vi "Fetch Array (Voltage).vi"(0 "VISA resource name":refnum<visa-resource-name>, 11 "error in (no error)":errorcluster) -> (4 "VISA resource name out":refnum<visa-resource-name>, 6 "Samples (V)":dbl[](array[numeric]), 15 "error out":errorcluster)   [LabVIEW 2012, in "NH Research Regenerative Test Series.lvlib"]
doc: "Return an array containing the instantaneous input voltage in Volts. Query Number of Samples is called internally to read how many samples are available to read from the instruments buffer.\n\nWaveforms are captured with every initiated measurement based on the Set Aperture Length.vi and Set Number of Samples.vi commands. A measurement must be initiated first using a Read command or calling Initiate Measurement.vi."
uses:
  <instrlib>/NH Research Regenerative Test Series/NH Research Regenerative Test Series.lvlib
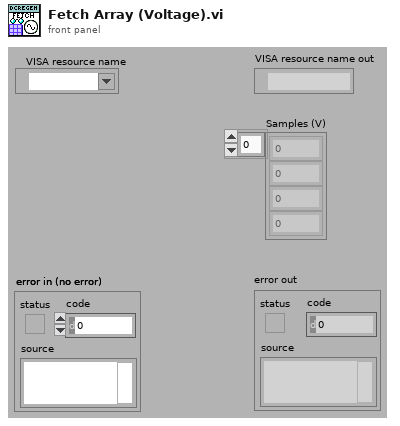
[diagram p1: front panel]
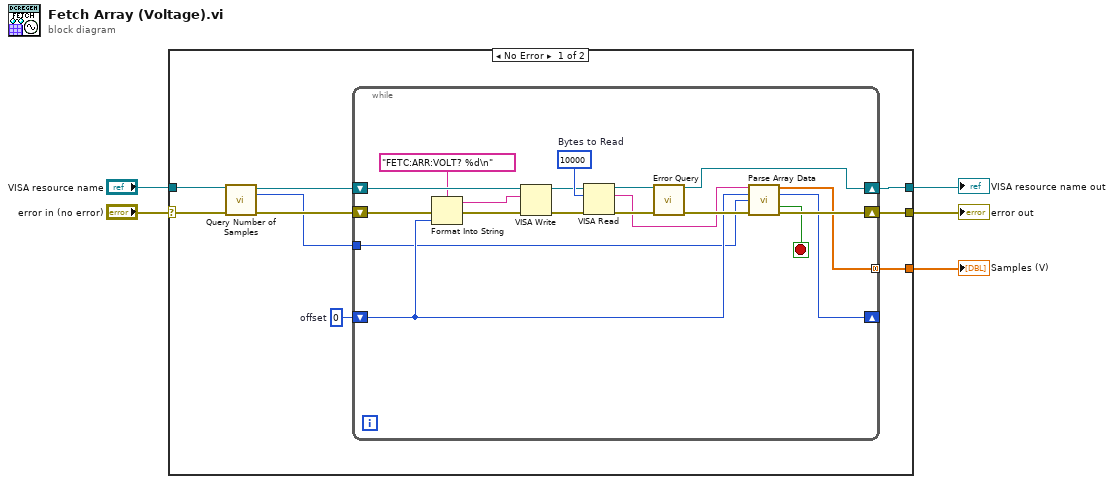
[diagram p0: block diagram]
diagram:
  n1 = case shown="No Error" "error in (no error)" {
    selector: "error in (no error)" -> [w10 w35]
    tunnel: [w13 w35] -> w4
    tunnel: [w14 w34] -> w1
    tunnel: "VISA resource name" -> [w9 w34]
    tunnel: [w12 _] -> w2
    frame No Error {
      w11 = 0  # offset
      n2 = call <instrlib>:"Query Number of Samples.vi"("VISA resource name"=w9, "error in (no error)"=w10) -> ("VISA resource name out"=w8:refnum<visa-resource-name>, "Number of Samples"=w6:u32, "error out"=w7:errorcluster)  [unwired: 11 in]
      n3 = while {
        shift-right: [w22] -> w13
        shift-left: w7 -> [w26]
        shift-right: [w15] -> w14
        shift-left: w8 -> [w30]
        tunnel: [w17] -> w12 mode=concatenating
        shift-right: [w18] -> _
        shift-left: w11 -> [w20]
        tunnel: w6 -> [w19]
        stop <- w16 stop-if-true
        w33 = u32 10000  # Bytes to Read
        n4 = Format Into String(format string="FETC:ARR:VOLT? %d\n", error in=w26, w20) -> (resulting string=w24:string, error out=w25:errorcluster)  [unwired: 1 in]
        n5 = VISA Write(VISA resource name=w30, write buffer=w24, error in (no error)=w25) -> (VISA resource name out=w31:refnum<visa-resource-name>, error out=w32:errorcluster)  [unwired: 1 out]
        n6 = VISA Read(VISA resource name=w31, byte count=w33, error in (no error)=w32) -> (VISA resource name out=w29:refnum<visa-resource-name>, read buffer=w21:string, error out=w28:errorcluster)  [unwired: 1 out]
        n7 = call <instrlib>:"Error Query.vi"("VISA resource name"=w29, "error in (no error)"=w28) -> ("VISA resource name out"=w15:refnum<visa-resource-name>, "error out"=w23:errorcluster)  [unwired: 10 in, 2 out]
        n8 = call <instrlib>:"Parse Array Data.vi"("Samples String"=w21, "Current Index"=w20, "Number of Samples"=w19, "error in (no error)"=w23) -> ("Samples"=w17:dbl[], "Next Index"=w18:i32, "Stop Reading Samples"=w16:bool, "error out"=w22:errorcluster)  [unwired: 8 in]
      }
    }
    frame Error {
    }
  }
  "error out" <- w4
  "VISA resource name out" <- w1
  "Samples (V)" <- w2
